vi "90_degree_turn.vi"(0 "Right?":bool, 1 "Speed (mm/s)":dbl) -> ()   [LabVIEW 2015]
uses:
  class/Car.lvclass
panel:
  out "Gyro Reading":dbl
  out "x > y?":bool
  in  "x > y? 2":bool
  out "Numeric":i32
  out "Integration Count":i32
  out "x+y":i32
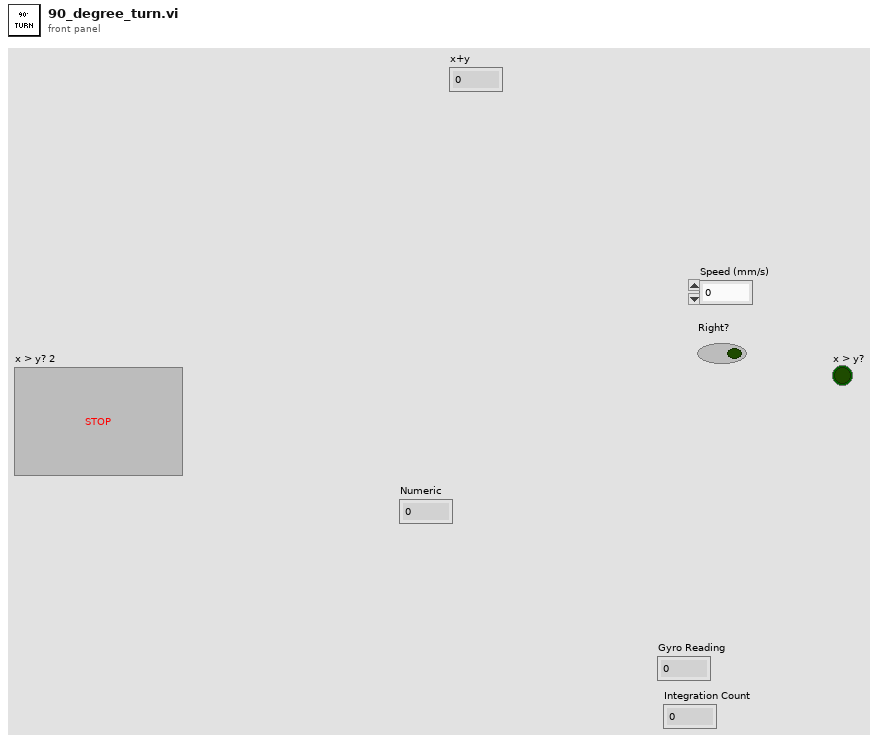
[diagram p1: front panel]
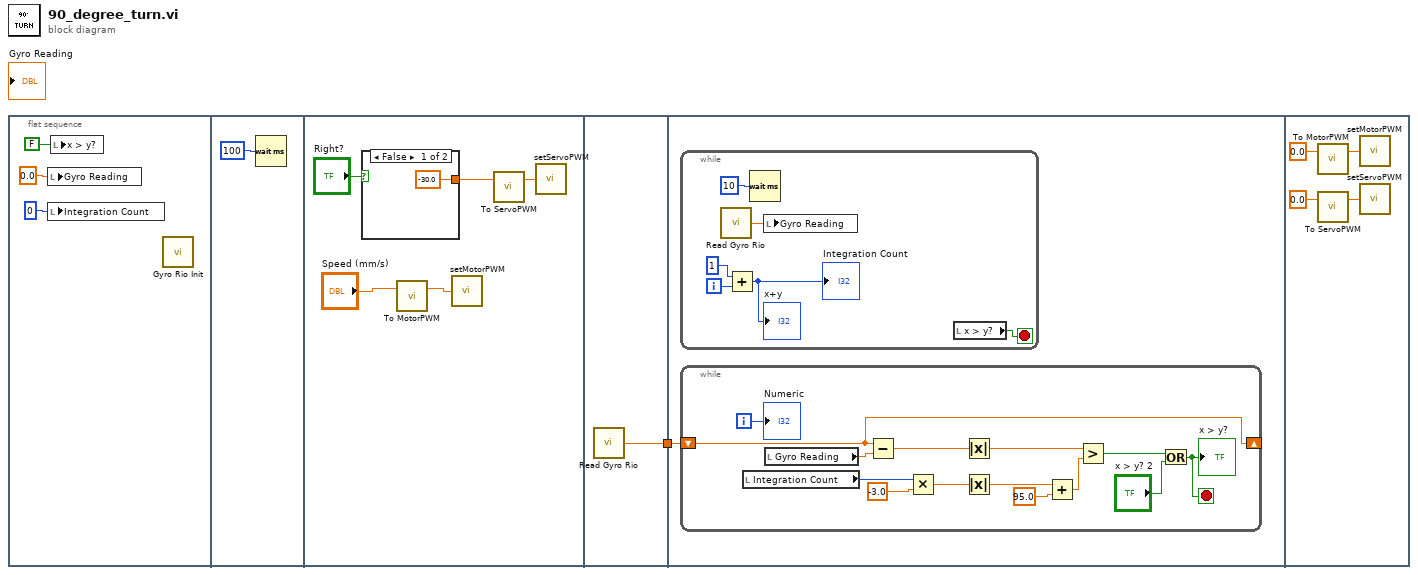
[diagram p0: block diagram]
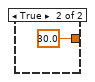
[diagram p2: hidden frame]
diagram:
  n1 = flat-sequence {
    tunnel: [w13] -> w1
    tunnel: w1 -> [w14]
    frame #0 {
      n2 = local write "Gyro Reading"(0.0 ("Gyro Reading")) -> ()
      n3 = local write "Integration Count"(0 ("Integration Count")) -> ()
      n4 = local write "x > y?"(FALSE) -> ()
      n5 = call "Gyro Rio Init.vi"() -> ()  [unwired: 12 in]
    }
    frame #1 {
      n6 = Wait (ms)(milliseconds to wait=u32 100) -> ()  [unwired: 1 out]
    }
    frame #2 {
      n7 = case shown="False" "Right?" {
        tunnel: [-30.0 30.0] -> w6
        frame False {
        }
        frame True {
        }
      }
      n8 = call "To MotorPWM.vi"("Speed"="Speed (mm/s)") -> ("MotorPWM"=w9:dbl)  [unwired: 1 in, 1 out]
      n9 = call "setMotorPWM.vi"("Numeric"=w9) -> ()
      n10 = call "To ServoPWM.vi"("Wheel Angle"=w6) -> ("ServoPWM"=w10:dbl)  [unwired: 1 in, 1 out]
      n11 = call "setServoPWM.vi"("Servo PWM"=w10) -> ()
    }
    frame #3 {
      n12 = call "Read Gyro Rio.vi"() -> ("integral y(t)"=w13:dbl)  [unwired: 1 in, 2 out]
    }
    frame #4 {
      n13 = while {
        i -> [w15]
        stop <- w17 stop-if-true
        n14 = call "Read Gyro Rio.vi"() -> ("integral y(t)"=w16:dbl)  [unwired: 1 in, 2 out]
        n15 = Add(x=1, y=w15) -> (x+y=→"Integration Count" →"x+y":i32)
        n16 = Wait (ms)(milliseconds to wait=u32 10) -> ()  [unwired: 1 out]
        n17 = local write "Gyro Reading"(w16) -> ()
        n18 = local read "x > y?"() -> (w17:bool)
      }
      n19 = while {
        shift-right: [w32] -> _
        shift-left: w14 -> [w32]
        i -> [w21]
        stop <- w22 stop-if-true
        n20 = local read "Integration Count"() -> (w29:i32)
        n21 = local read "Gyro Reading"() -> (w31:dbl)
        n22 = Subtract(x=w32, y=w31) -> (x-y=w33:dbl)
        n23 = Multiply(x=w29, y=-3.0) -> (x*y=w27:dbl)
        n24 = Absolute Value(x=w33) -> (abs(x)=w34:dbl)
        n25 = Absolute Value(x=w27) -> (abs(x)=w30:dbl)
        n26 = Add(x=w30, y=95.0) -> (x+y=w25:dbl)
        n27 = Greater?(x=w34, y=w25) -> (0:w24:bool)
        n28 = Or(x=w24, y="x > y? 2") -> (x .or. y?=w22:bool)
        "x > y?" <- w22
        "Numeric" <- w21
      }
    }
    frame #5 {
      n29 = call "To MotorPWM.vi"("Speed"=0.0) -> ("MotorPWM"=w35:dbl)  [unwired: 1 in, 1 out]
      n30 = call "To ServoPWM.vi"("Wheel Angle"=0.0) -> ("ServoPWM"=w37:dbl)  [unwired: 1 in, 1 out]
      n31 = call "setMotorPWM.vi"("Numeric"=w35) -> ()
      n32 = call "setServoPWM.vi"("Servo PWM"=w37) -> ()
    }
  }
